vi "Kalman Filter Step.vi"(9 "Control Input":T1, 10 "Observations":T1, 11 "Kalman Filter In":T2) -> (3 "Kalman Filter Out":T2)   [LabVIEW 2020]
uses:
  ctl/Kalman Filter Instance.ctl
  <vilib>/Analysis/Matrix/Datatypes/RealMatrix.ctl
  ctl/Dynamical System Matrices.ctl
  <vilib>/Analysis/Matrix/NI_Matrix.lvlib
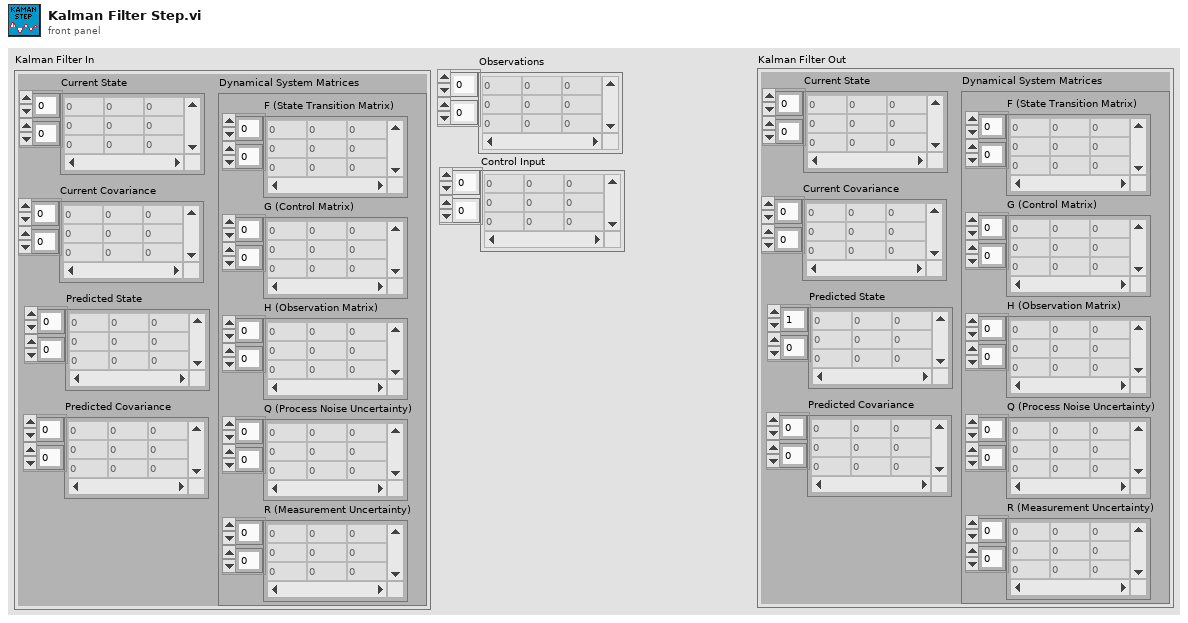
[diagram p1: front panel]
types:
  T1 = typedef "NI_Matrix.lvlib/RealMatrix.ctl" = dbl[][]
  T2 = typedef "Kalman Filter Instance.ctl" = cluster{"Current State":T1, "Current Covariance":T1, "Predicted State":T1, "Predicted Covariance":T1, "Dynamical System Matrices":T3}
  T3 = typedef "Dynamical System Matrices.ctl" = cluster{"F (State Transition Matrix)":T1, "G (Control Matrix)":T1, "H (Observation Matrix)":T1, "Q (Process Noise Uncertainty)":T1, "R (Measurement Uncertainty)":T1}
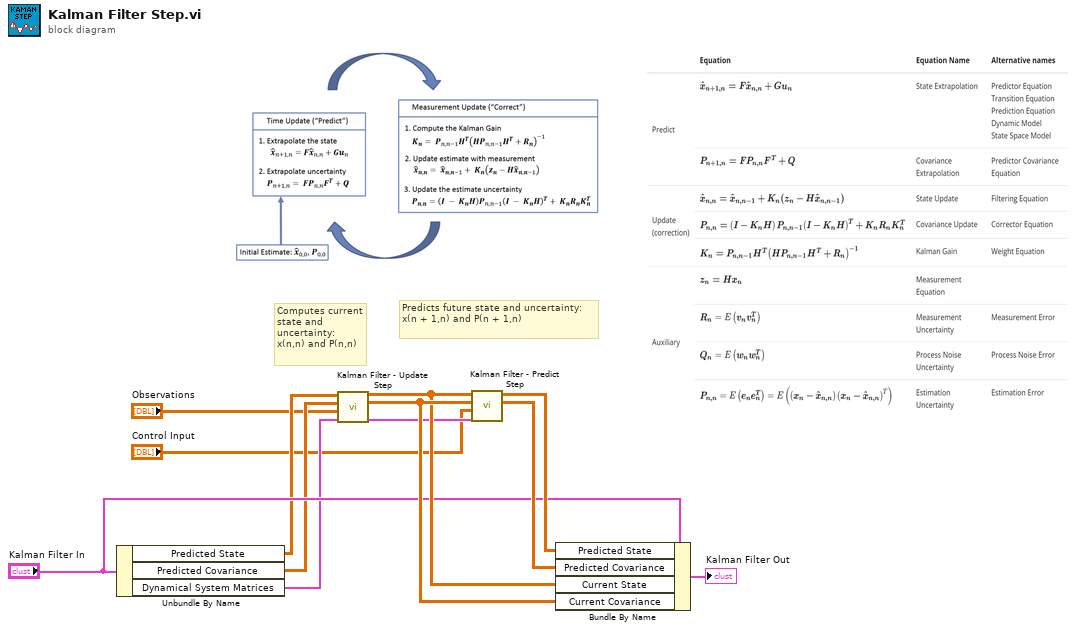
[diagram p0: block diagram]
diagram:
  # "Predicts future state and uncertainty: x(n + 1,n) and P(n + 1,n)"
  # "Computes current state and uncertainty: x(n,n) and P(n,n)"
  n1 = Unbundle By Name("Kalman Filter In") -> ("Predicted State"=w4:T1, "Predicted Covariance"=w5:T1, "Dynamical System Matrices"=w3:T3)
  n2 = call "Kalman Filter - Update Step.vi"("Dynamical System Matrices In"=w3, "Observations"="Observations", "Old Covariance"=w5, "Old State"=w4) -> ("Dynamical System Matrices Out"=w6:T3, "Updated Covariance"=w9:T1, "Updated State"=w8:T1)  [unwired: 5 in]
  n3 = call "Kalman Filter - Predict Step.vi"("Dynamical System Matrices In"=w6, "Control Input"="Control Input", "Initial Covariance"=w9, "Initial State"=w8) -> ("Predicted Covariance"=w11:T1, "Predicted State"=w10:T1)  [unwired: 5 in, 1 out]
  n4 = Bundle By Name(cluster="Kalman Filter In", "Predicted State"=w10, "Predicted Covariance"=w11, "Current State"=w8, "Current Covariance"=w9) -> (→"Kalman Filter Out":T2)
